vi "Frame Size.vi"() -> (3 "Frame Size":i32)   [LabVIEW 2018, in "OOPanel.lvlib" / "PanelArray.lvclass"]
uses:
  PanelArray.lvclass
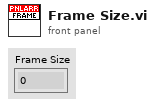
[diagram p1: front panel]
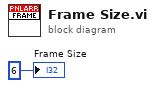
[diagram p0: block diagram]
diagram:
  "Frame Size" <- 6 ("Frame Size")
